vi "CLD 15 FGV for Text String Parsing Exercise.vi"(8 "Error In":errorcluster, 11 "Mode":T2) -> (0 "Error Out":errorcluster)   [LabVIEW 2009]
doc: "CLD 15 This VI reads the file and uses two subVI's to parse then format the file data for use."
uses:
  CLD 15 CSV file data structure.ctl
  CLD 15 CSV file enum.ctl
panel:
  out "Formatted Data Out":T1[](array[typedef])
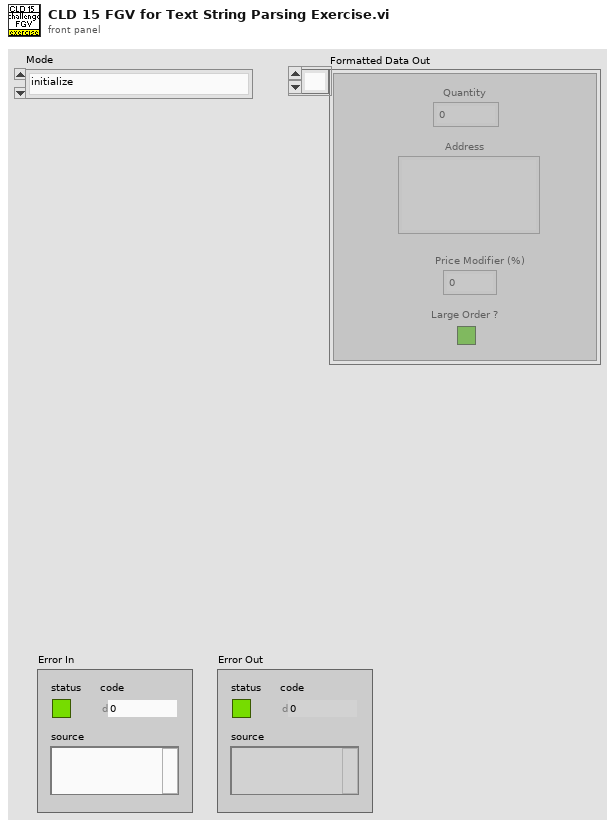
[diagram p1: front panel]
types:
  T1 = typedef "CLD 15 CSV file data structure.ctl" = cluster{"Quantity":i32, "Address":string, "Price Modifier (%)":dbl, "Large Order ?":bool}
  T2 = typedef "CLD 15 CSV file enum.ctl" = enum16{"initialize", "Read CSV", "Process Data", "Write CSV"}
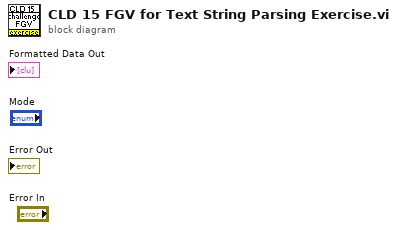
[diagram p0: block diagram]
diagram:
